vi "PH_IEEE1394Camera.evt call Connect.vi"(0 "i ref in":refnum<vi>, 2 "Instance":string, 4 "Cam Name":string="N/A", 5 "error in (no error)":errorcluster) -> (14 "i ref out":refnum<vi>, 19 "error out":errorcluster)   [LabVIEW 2014]
doc: "This VI sends a simple call for Connect."
uses:
  CSCore/CSSystem/CoreLib/CoreLib.string 2 byte array.vi
  CSCore/CSSystem/CoreLib/CoreLib.lvlib
  CSCore/BaseProcess/BaseProcess.lvlib
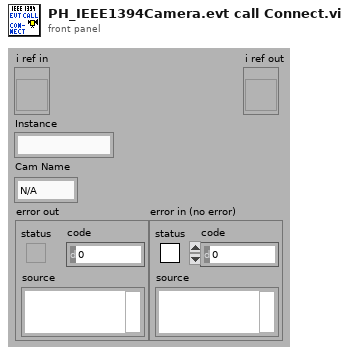
[diagram p1: front panel]
types:
  T1 = typedef "CoreDefs.rawDataType.ctl" = i8[]
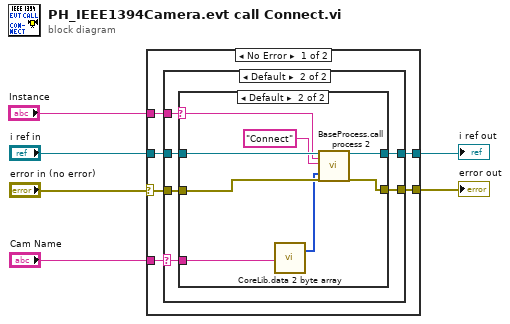
[diagram p0: block diagram]
diagram:
  n1 = case shown="No Error" "error in (no error)" {
    selector: "error in (no error)" -> [w9 w31]
    tunnel: [w12 w32] -> w3
    tunnel: [w11 w31] -> w2
    tunnel: "i ref in" -> [w10 w32]
    tunnel: "Instance" -> [w8 _]
    tunnel: "Cam Name" -> [w7 _]
    frame No Error {
      n2 = case shown="Default" w7 {
        selector: w7 -> [_ w15]
        tunnel: [w14 w20] -> w12
        tunnel: [w13 w19] -> w11
        tunnel: w10 -> [w14 w18]
        tunnel: w9 -> [w13 w17]
        tunnel: w8 -> [_ w16]
        frame "", "N/A" {
        }
        frame Default {
          n3 = case shown="Default" w16 {
            selector: w16 -> [_ w23]
            tunnel: [w22 w30] -> w20
            tunnel: [w21 w29] -> w19
            tunnel: w18 -> [w22 w28]
            tunnel: w17 -> [w21 w26]
            tunnel: w15 -> [_ w25]
            frame "N/A" {
            }
            frame Default {
              n4 = call-poly "CoreLib.data 2 byte array.vi"("string"=w25) -> ("byteArray out"=w24:T1)  [unwired: 18 in]
              n5 = call "BaseProcess.call process 2.vi"("i ref in"=w28, "Object"=w23, "Selector"="Connect", "Data"=w24, "error in (no error)"=w26) -> ("i ref out"=w30:refnum<vi>, "error out"=w29:errorcluster)  [unwired: 13 in]
            }
          }
        }
      }
    }
    frame Error {
    }
  }
  "error out" <- w2
  "i ref out" <- w3
